vi "Load-FPGA.vi"(8 "Error In":errorcluster) -> (0 "Error Out":errorcluster)   [LabVIEW 2019]
uses:
  <vilib>/FPGAPlugInAG/myRIO-1900/niLvFpga_Open_myRIO-1900.vi
  <vilib>/rvi/interface/common/dynamic/niFpgaDynamicAddResources.vi
  <vilib>/myRIO/Common/Instrument Driver Framework/Utilities/vis/FPGA Ref Manager.vi
  <vilib>/Utility/error.llb/Error Cluster From Error Code.vi
  <vilib>/myRIO/Common/Instrument Driver Framework/Utilities/vis/Ref Counter.vi
  <vilib>/FPGAPlugInAG/Dynamic/niLvFpga_Run_Dynamic.vi
  Variable/FPGA-Referense.vi
  <vilib>/rvi/interface/nirviOpenFPGA/nirviOpenFPGA.xnode
  FPGA/FPGA Bitfiles/FPGAEncoderError_FPGATarget_FPGAMainDefault_e7UsQj9JDpI.lvbitx
  <vilib>/rvi/interface/nirviMethod/nirviMethod.xnode
  <vilib>/myRIO/Instrument Drivers/Utilities/Utilities.lvlib
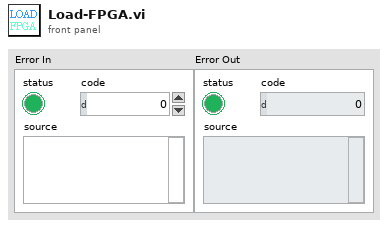
[diagram p1: front panel]
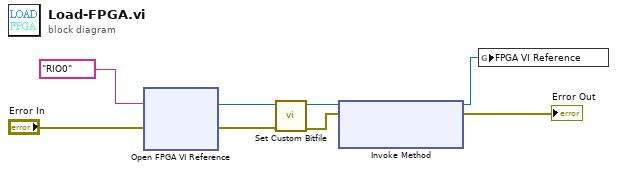
[diagram p0: block diagram]
diagram:
  n1 = xnode "Open FPGA VI Reference"("error in"="Error In", "resource name"=tag "RIO0") -> ("FPGA VI Reference Out"=w3:refnum<k20>, "error out"=w2:errorcluster)
  n2 = call <vilib>:"Set Custom Bitfile.vi"("error in (no error)"=w2, "Custom FPGA Reference In"=w3) -> ("error out"=w4:errorcluster, "Custom FPGA Reference Out"=w5:refnum<k20>)  [unwired: 8 in]
  n3 = xnode "Invoke Method"("FPGA VI Reference In"=w5, "error in"=w4) -> ("FPGA VI Reference Out"=w1:refnum<k20>, "error out"=→"Error Out":errorcluster)  [unwired: 1 in]
  n4 = global write "FPGA-Referense.vi" "FPGA VI Reference"(w1) -> ()
